vi "GetSetTimeLeft.vi"(0 "VISA resource name":refnum<visa-resource-name>, 1 "get/set":T3=enum."set", 2 "Time input cluster":T1 {"Seconds\n(0-359999)" max=359999 step=1; "Minutes\n(0-5999)" max=5999 step=1; "Hours\n(0-99)" max=99 step=1}, 5 "error in":errorcluster) -> (14 "VISA resource name out":refnum<visa-resource-name>, 15 "Time left string":string, 16 "Time left cluster":T2, 19 "error out":errorcluster)   [LabVIEW 2023, in "Thermotron 8800.lvlib"]
doc: "TLFT\nCommand name: Send or load time left\nCommand type: Program status; edit from hold\nDescription: Queries the 8800 for the time left in the current interval. The edit from hold operation command temporarily changes the current interval’s time left counter.\nSyntax: TLFT? or TLFThh:mm:ss\nWhere hh is hours, mm is minutes, and ss is seconds.\nData type: String\nQuery example: TLFT?\n8800 response: 1:17:57 (The time left in the current interval is 1 hour, 17 minutes, 57 seconds.)\nOperation example: TLFT::85\n8800 response: This command sets the time left in the current interval to 1 minute, 25 seconds."
uses:
  Thermotron 8800.lvlib
  Private/get set.ctl
panel:
  # ":"
  # ":"
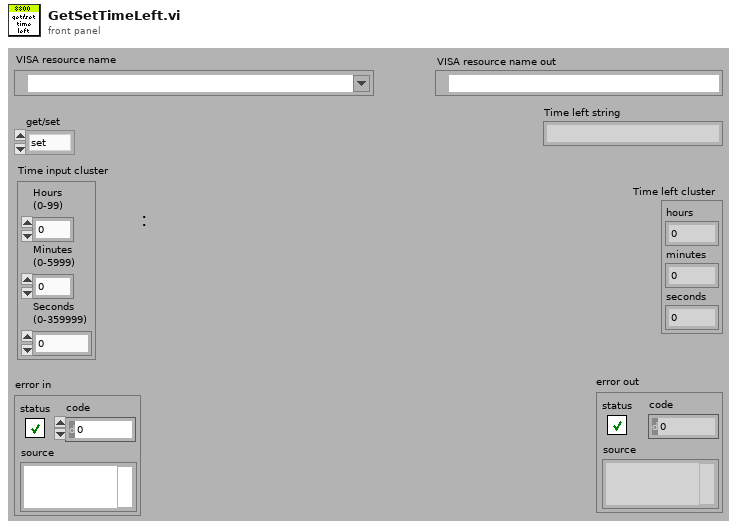
[diagram p1: front panel]
types:
  T1 = cluster{"Hours\n(0-99)":u8, "Minutes\n(0-5999)":u16, "Seconds\n(0-359999)":u32}
  T2 = cluster{"hours":i32, "minutes":i32, "seconds":i32}
  T3 = typedef "Thermotron 8800.lvlib/get set.ctl" = enum16{"get", "set"}
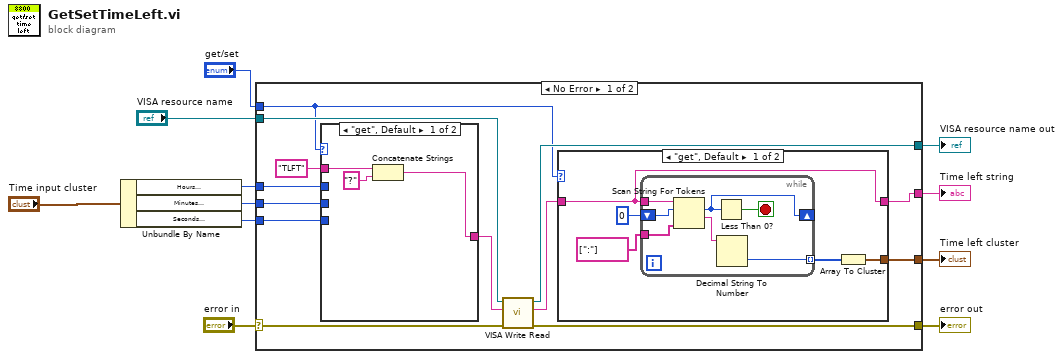
[diagram p0: block diagram]
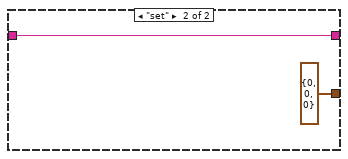
[diagram p2: hidden frame]
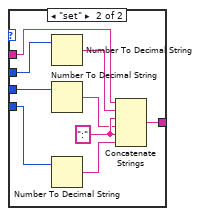
[diagram p3: hidden frame]
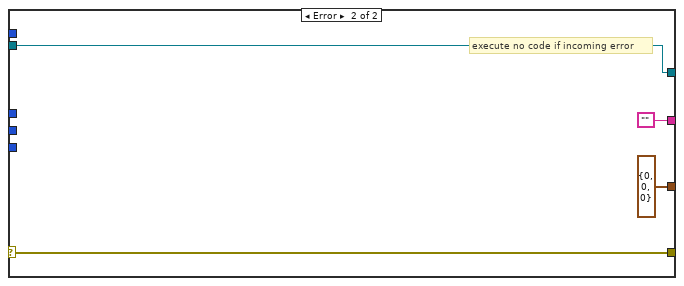
[diagram p4: hidden frame]
diagram:
  n1 = Unbundle By Name("Time input cluster") -> ("Hours\n(0-99)"=w3:u8, "Minutes\n(0-5999)"=w2:u16, "Seconds\n(0-359999)"=w1:u32)
  n2 = case shown="No Error" "error in" {
    selector: "error in" -> [w20 w54]
    tunnel: [w23 w54] -> w11
    tunnel: [w22 w53] -> w10
    tunnel: "VISA resource name" -> [w21 w53]
    tunnel: "get/set" -> [w15 _]
    tunnel: [w13 ""] -> w7
    tunnel: w3 -> [w19 _]
    tunnel: w2 -> [w17 _]
    tunnel: w1 -> [w16 _]
    tunnel: [w12 cluster{"[0]":i32, "[1]":i32, "[2]":i32} {"[0]"=0, "[1]"=0, "[2]"=0}] -> w5
    frame No Error {
      n3 = case shown="\"get\", Default" w15 {
        tunnel: [w41 w50] -> w24
        tunnel: w19 -> [_ w49]
        tunnel: "TLFT" ("8800 Command") -> [w39 w48]
        tunnel: w17 -> [_ w45]
        tunnel: w16 -> [_ w43]
        frame "get", Default {
          n4 = Concatenate Strings(w39, "?" ("8800 Command")) -> (w41:string)
        }
        frame "set" {
          w46 = ":" ("string")
          n5 = Number To Decimal String(number=w49) -> (decimal integer string=w47:string)  [unwired: 1 in]
          n6 = Number To Decimal String(number=w45) -> (decimal integer string=w44:string)  [unwired: 1 in]
          n7 = Number To Decimal String(number=w43) -> (decimal integer string=w42:string)  [unwired: 1 in]
          n8 = Concatenate Strings(w48, w47, w46, w44, w46, w42) -> (w50:string)
        }
      }
      n9 = call "VISA Write Read.vi"("error in (no error)"=w20, "8800 Command"=w24, "VISA Refnum in"=w21) -> ("error out"=w23:errorcluster, "read buffer"=w14:string, "VISA Refnum out"=w22:refnum<visa-resource-name>)  [unwired: 6 in]
      n10 = case shown="\"get\", Default" w15 {
        tunnel: w14 -> [w25 w38]
        tunnel: [w25 w38] -> w13
        tunnel: [w26 cluster{"[0]":i32, "[1]":i32, "[2]":i32} {"[0]"=0, "[1]"=0, "[2]"=0}] -> w12
        frame "get", Default {
          n11 = while {
            tunnel: string[] [":"] ("delimiters (\\s,\\t,\\r,\\n)") -> [w35]
            tunnel: w25 -> [w36]
            shift-right: [w32] -> _
            shift-left: 0 ("offset") -> [w34]
            tunnel: [w30] -> w27 mode=indexing
            stop <- w33 stop-if-true
            n12 = Scan String For Tokens(6:w35, 8:w34, 9:w36) -> (1:w31:string, 2:w32:i32)  [unwired: 3 in, 2 out]
            n13 = Less Than 0?(x=w32) -> (x < 0?=w33:bool)
            n14 = Decimal String To Number(string=w31) -> (number=w30:i32)  [unwired: 2 in, 1 out]
          }
          n15 = Array To Cluster(array=w27) -> (cluster=w26:cluster{"[0]":i32, "[1]":i32, "[2]":i32})
        }
        frame "set" {
        }
      }
    }
    frame Error {
      # "execute no code if incoming error"
    }
  }
  "VISA resource name out" <- w10
  "error out" <- w11
  "Time left string" <- w7
  "Time left cluster" <- w5
